vi "Generic Request.vi"   [LabVIEW 2020, in "Library Commun.lvlib" / "Library Http.lvlib" / "Session.lvclass"]
doc: "Sends a web request that submits data or a file to a server, web page, or web service. This VI uses the HTTP method specified by the <b>method</b> input."
uses:
  Session.lvclass
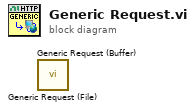
[diagram p0: block diagram]
diagram:
  n1 = call "Generic Request (File).vi"() -> ()  [unwired: 7 in, 5 out]
  n2 = call "Generic Request (Buffer).vi"() -> ()  [unwired: 7 in, 5 out]
